vi "Receive DBL.vi"(8 "error in (no error)":errorcluster, 10 "Broadcast DBL Msg":refnum<class "Broadcast DBL Msg.lvclass">, 11 "TopLevelApplication In":refnum<class "TopLevelApplication.lvclass">) -> (0 "error out":errorcluster, 3 "TopLevelApplication Out":refnum<class "TopLevelApplication.lvclass">)   [LabVIEW 2015, in "TopLevelApplication.lvlib" / "TopLevelApplication.lvclass"]
uses:
  TopLevelApplication.lvclass
  IViewable/IViewable Messages/Broadcast DBL Msg/Broadcast DBL Msg.lvclass
  IViewable/IViewable Messages/Broadcast DBL Msg/Broadcast DBL Msg.lvclass/Broadcast DBL Msg.ctl
  Dialog Box Implementations/OneButtonDialogBox/OneButtonDialogBox.lvclass
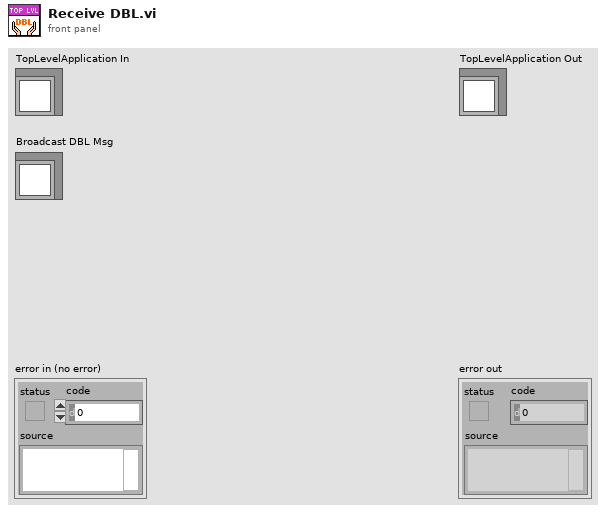
[diagram p1: front panel]
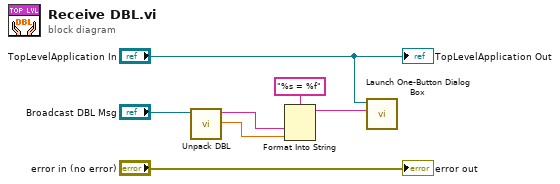
[diagram p0: block diagram]
diagram:
  n1 = call "Unpack DBL.vi"("Broadcast DBL Msg In"="Broadcast DBL Msg") -> ("Value"=w4:dbl, "Name"=w5:string)  [unwired: 9 in]
  n2 = Format Into String(format string="%s = %f", w5, w4) -> (resulting string=w2:string)  [unwired: 2 in, 1 out]
  n3 = call "Launch One-Button Dialog Box.vi"("Message Text"=w2, "Dialog Launcher"="TopLevelApplication In") -> ()  [unwired: 9 in, 1 out]
  "error out" <- "error in (no error)"
  "TopLevelApplication Out" <- "TopLevelApplication In"
